vi "Pracownia3.vi"() -> ()   [LabVIEW 2023]
panel:
  out "y":string
  out "y":string
  out "y":dbl
  in  "stop":bool
  in  "Enum":T1(ring)
  in  "c":dbl
  in  "b":dbl
  in  "a":dbl
  in  "x":dbl
  in  "?":bool
  # "y = a + bx + cx^2"
  # "y =a + bx^2 - 3x^4"
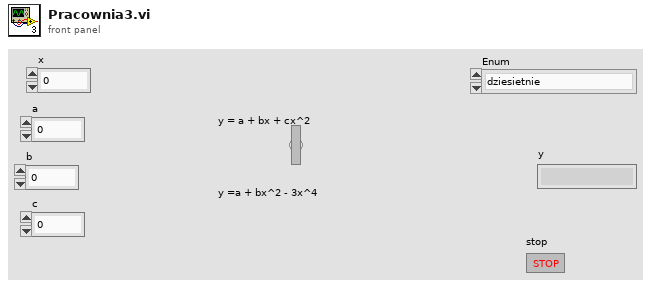
[diagram p1: front panel]
types:
  T1 = enum16{"dziesietnie", "ósemkowo", "szesnastkowo"}
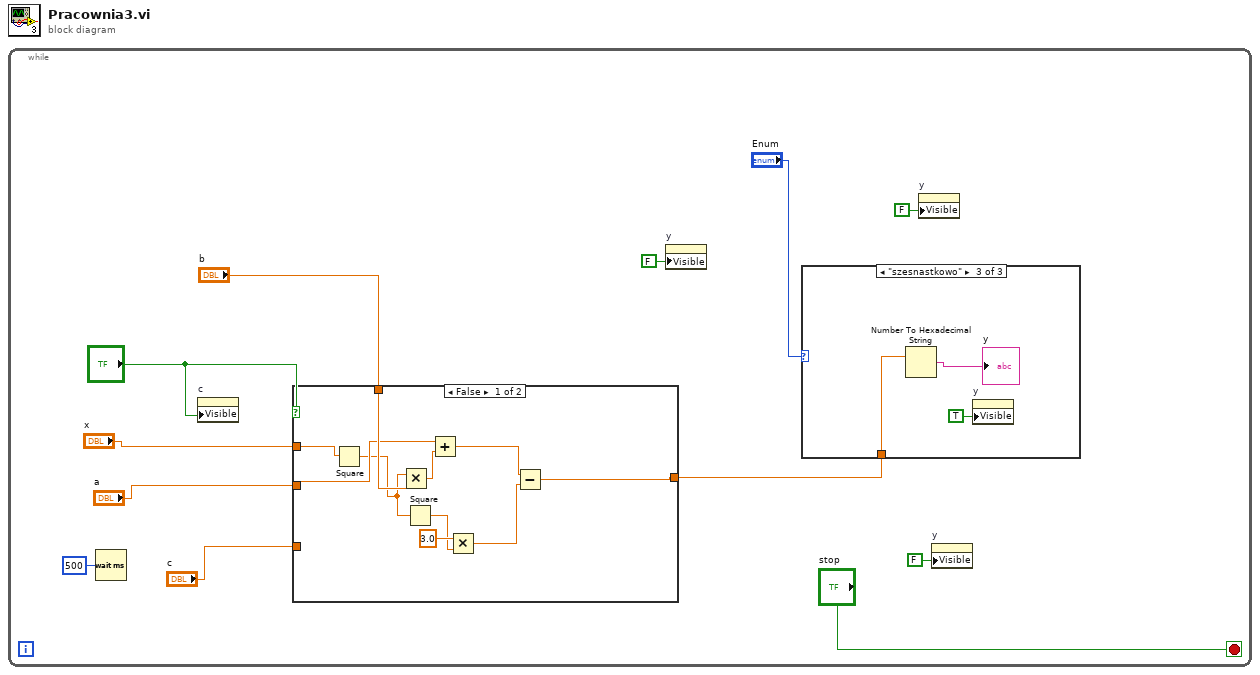
[diagram p0: block diagram]
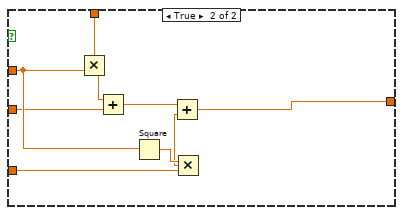
[diagram p2: hidden frame]
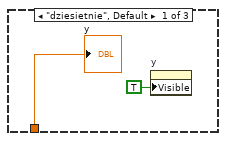
[diagram p3: hidden frame]
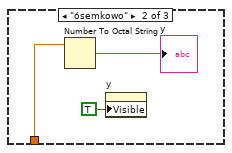
[diagram p4: hidden frame]
diagram:
  n1 = while {
    stop <- "stop" stop-if-true
    n2 = Wait (ms)(milliseconds to wait=u32 500) -> ()  [unwired: 1 out]
    n3 = property on="c" class="DigNum (strict)"("Visible"="?") -> ()  [unwired: 2 in, 2 out]
    n4 = case shown="False" "?" {
      tunnel: "b" -> [w21 w27]
      tunnel: "x" -> [w22 w26]
      tunnel: "a" -> [w20 w25]
      tunnel: "c" -> [_ w24]
      tunnel: [w13 w23] -> w4
      frame False {
        n5 = Square(x=w22) -> (x^2=w16:dbl)
        n6 = Multiply(x=w16, y=w21) -> (x*y=w19:dbl)
        n7 = Square(x=w16) -> (x^2=w15:dbl)
        n8 = Add(x=w20, y=w19) -> (x+y=w18:dbl)
        n9 = Multiply(x=3.0, y=w15) -> (x*y=w14:dbl)
        n10 = Subtract(x=w18, y=w14) -> (x-y=w13:dbl)
      }
      frame True {
        n11 = Multiply(x=w27, y=w26) -> (x*y=w31:dbl)
        n12 = Add(x=w31, y=w25) -> (x+y=w29:dbl)
        n13 = Square(x=w26) -> (x^2=w30:dbl)
        n14 = Multiply(x=w30, y=w24) -> (x*y=w28:dbl)
        n15 = Add(x=w29, y=w28) -> (x+y=w23:dbl)
      }
    }
    n16 = property on="y" class="DigNum (strict)"("Visible"=FALSE) -> ()  [unwired: 2 in, 2 out]
    n17 = case shown="\"szesnastkowo\"" "Enum" {
      tunnel: w4 -> [w33 w36 w39]
      frame "dziesietnie", Default {
        n18 = property on="y" class="DigNum (strict)"("Visible"=TRUE) -> ()  [unwired: 2 in, 2 out]
        "y" <- w33
      }
      frame "ósemkowo" {
        n19 = Number To Octal String(2:w36) -> (0:→"y":string)  [unwired: 1 in]
        n20 = property on="y" class="Str"("Visible"=TRUE) -> ()  [unwired: 2 in, 2 out]
      }
      frame "szesnastkowo" {
        n21 = Number To Hexadecimal String(2:w39) -> (0:→"y":string)  [unwired: 1 in]
        n22 = property on="y" class="Str"("Visible"=TRUE) -> ()  [unwired: 2 in, 2 out]
      }
    }
    n23 = property on="y" class="Str"("Visible"=FALSE) -> ()  [unwired: 2 in, 2 out]
    n24 = property on="y" class="Str"("Visible"=FALSE) -> ()  [unwired: 2 in, 2 out]
  }
